vi "Emballage_DefinirImprimanteParDefaut.vi"(8 "Error in":errorcluster caption="Error in (no error)", 11 "Imprimante":string) -> (0 "Error out":errorcluster)   [LabVIEW 2020]
panel:
  out "standard error":string caption="erreur standard"
  out "standard output":string caption="sortie standard"
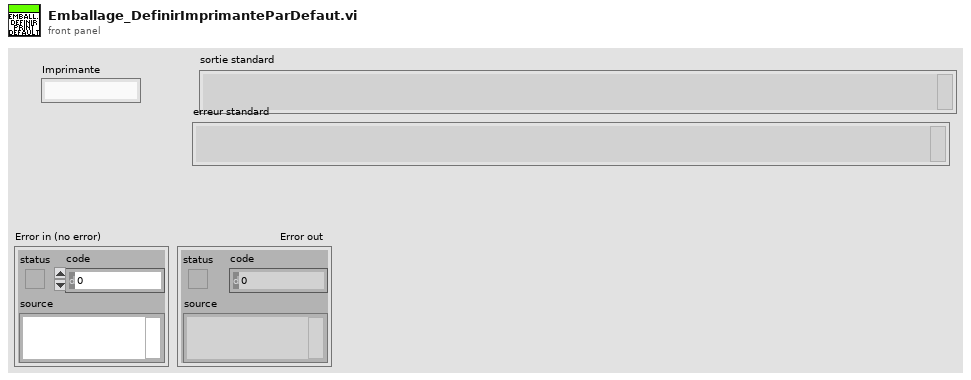
[diagram p1: front panel]
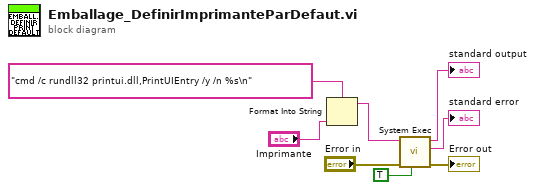
[diagram p0: block diagram]
diagram:
  n1 = Format Into String(format string="cmd /c rundll32 printui.dll,PrintUIEntry /y /n %s\n" ("command line"), "Imprimante") -> (resulting string=w2:string)  [unwired: 2 in, 1 out]
  n2 = call <vilib>:"System Exec.vi"("run minimized? (F)"=TRUE, "error in (no error)"="Error in", "command line"=w2) -> ("error out"=→"Error out":errorcluster, "standard error"=→"standard error":string, "standard output"=→"standard output":string)  [unwired: 5 in, 1 out]
